vi "ExtractHTMLSection.vi"(10 "Section":string, 11 "HTMLString":string) -> (3 "Extracted Section":string[](array[string]))   [LabVIEW 2020, in "StashRoyale.lvclass"]
uses:
  StashRoyale.lvclass
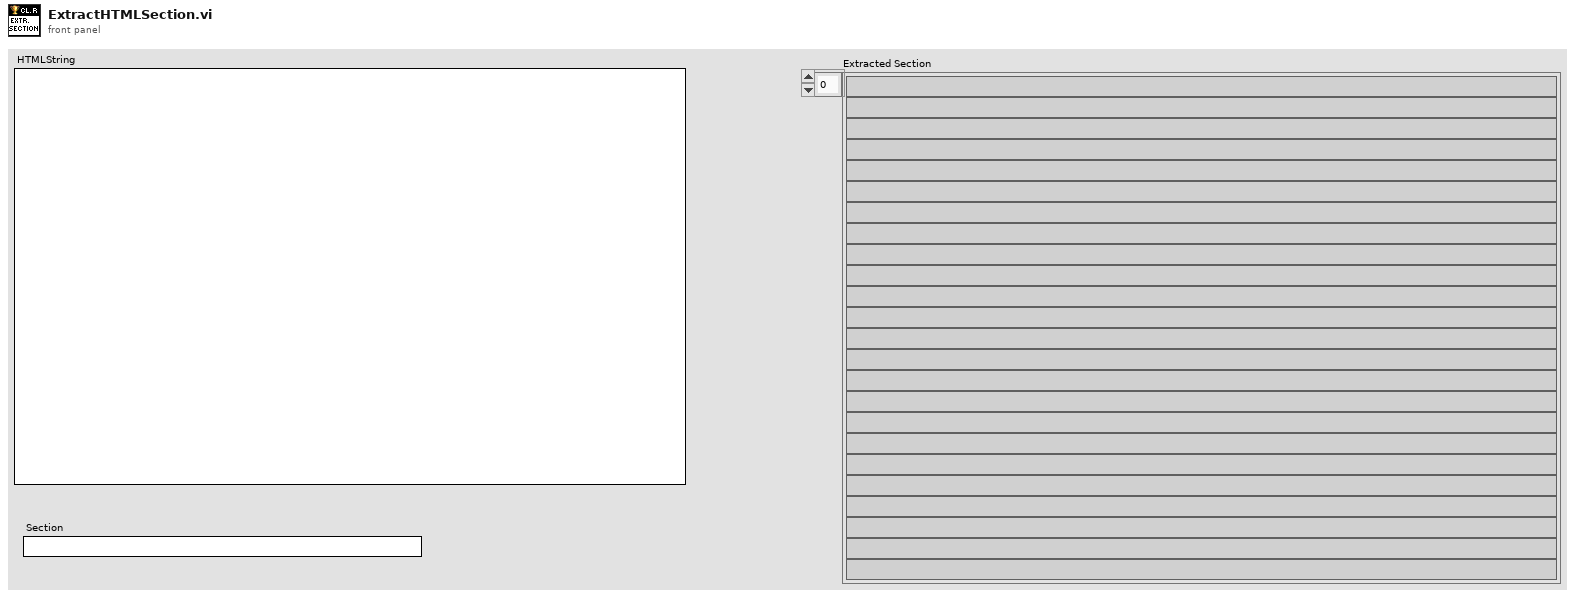
[diagram p1: front panel]
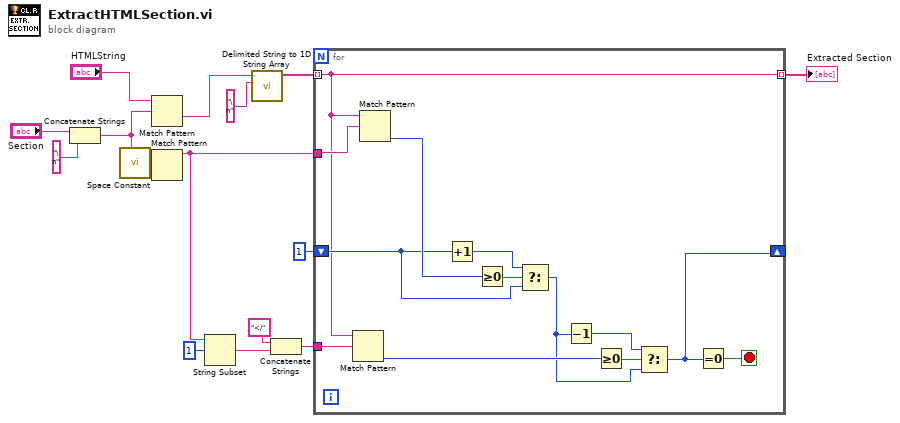
[diagram p0: block diagram]
diagram:
  n1 = Concatenate Strings("Section", "\n" ("string")) -> (w2:string)
  n2 = call <vilib>:"Space Constant.vi"() -> ("String"=w15:string)
  n3 = Match Pattern(string="HTMLString", regular expression=w2) -> (after substring=w12:string)  [unwired: 1 in, 3 out]
  n4 = Match Pattern(string=w2, regular expression=w15) -> (before substring=w9:string)  [unwired: 1 in, 3 out]
  n5 = String Subset(string=w9, offset (0)=1) -> (substring=w7:string)  [unwired: 1 in]
  n6 = call <vilib>:"Delimited String to 1D String Array.vi"("delimiter"="\n", "delimited string"=w12) -> ("string array"=w10:string[])  [unwired: 9 in]
  n7 = Concatenate Strings("</" ("string"), w7) -> (w6:string)
  n8 = for {
    tunnel: w9 -> [w28]
    tunnel: w10 -> [w17] mode=indexing
    tunnel: w6 -> [w27]
    shift-right: [w18] -> _
    shift-left: 1 -> [w23]
    tunnel: [w17] -> w3 mode=indexing
    stop <- w16 stop-if-true
    n9 = Match Pattern(string=w17, regular expression=w27) -> (offset past match=w20:i32)  [unwired: 1 in, 3 out]
    n10 = Match Pattern(string=w17, regular expression=w28) -> (offset past match=w24:i32)  [unwired: 1 in, 3 out]
    n11 = Increment(x=w23) -> (x+1=w25:i32)
    n12 = Greater Or Equal To 0?(x=w24) -> (x >= 0?=w26:bool)
    n13 = Select(t=w25, s=w26, f=w23) -> (s? t:f=w19:i32)
    n14 = Decrement(x=w19) -> (x-1=w22:i32)
    n15 = Greater Or Equal To 0?(x=w20) -> (x >= 0?=w21:bool)
    n16 = Select(t=w22, s=w21, f=w19) -> (s? t:f=w18:i32)
    n17 = Equal To 0?(x=w18) -> (x = 0?=w16:bool)
  }
  "Extracted Section" <- w3
